vi "Magnet Device (Set).vi"(6 "ISOBUS address":T8=-1 caption="ISOBUS address (-1)", 8 "error in":errorcluster, 10 "Magnet PSU":T3={"Nickname"="", "Bipolar Output"="", "Out Config"="SERS", "Current Limit"=0.0, "AtoB"=0.0, "Inductance"=0.0, "Switch Present"="", "Swh Htr Current"=0.0, "SW VLIM"=0.0, "Ignore Voltage Transient"="", "V Trans Time"=0.0, "Magnet PSU Signals"={"Target Current"=0.0, "Target Field"=0.0, "Target Current Rate"=0.0, "Target Field Rate"=0.0, "Switch Heater Status"="", "Set Switch Heater"="", "PSU Act Stat"="HOLD"}} {"Magnet PSU Signals"."Target Field Rate" min=0.0 max=50.0 step=0.01 format="%#.2f"; "Magnet PSU Signals"."Target Current Rate" min=0.0 max=1200.0 step=0.01 format="%#.2f"; "Magnet PSU Signals"."Target Field" min=-360.0 max=360.0 step=0.01 format="%#.2f"; "Magnet PSU Signals"."Target Current" min=-360.0 max=360.0 step=0.01 format="%#.2f"; "V Trans Time" min=0.0 max=120.0 step=0.01 format="%#.2f"; "SW VLIM" min=0.0 max=12.49 step=0.01 format="%#.2f"; "Swh Htr Current" min=0.0 max=125.0 step=0.01 format="%#.2f"; "Inductance" min=1.0 max=500.0 step=0.01 format="%#.2f"; "AtoB" min=1.0 max=30.0 step=0.01 format="%#.2f"; "Current Limit" min=0.0 max=360.0 step=0.01 format="%#.2f"}, 11 "Mercury Reference In":T9) -> (0 "error out":errorcluster, 2 "Response":T1, 3 "Mercury Reference Out":T9, 4 "Valid?":T2)   [LabVIEW 2013, in "Mercury iXX.lvlib" / "Magnet.lvlib"]
doc: "Set the auxiliary device configuration."
uses:
  Magnet.lvlib
  Mercury iXX.lvlib
  Private/Controls/Command Verbs.ctl
  Controls/Comms Transport Layer.ctl
  Controls/Mercury Reference.ctl
  Controls/Is Valid LED.ctl
  Controls/Response String.ctl
  Controls/ISOBus Address.ctl
  Private/Controls/Query Dynamic Reference.ctl
  Controls/Output Configuration.ctl
  Controls/Switch Heater.ctl
  Controls/PSU Actions.ctl
  Controls/Signals (Set).ctl
  Controls/Device (Set).ctl
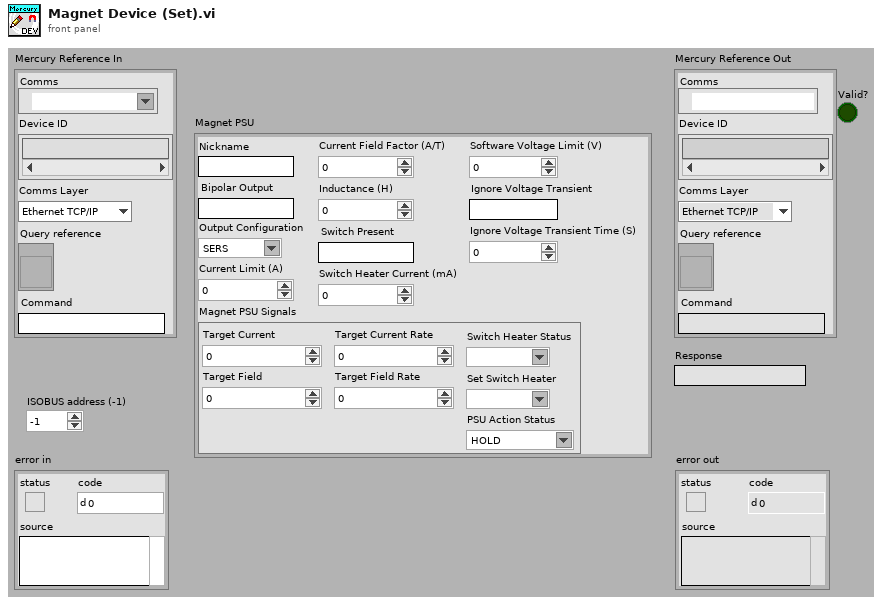
[diagram p1: front panel]
types:
  T1 = typedef "Mercury iXX.lvlib/Response String.ctl" = string
  T2 = typedef "Mercury iXX.lvlib/Is Valid LED.ctl" = bool
  T3 = typedef "Mercury iXX.lvlib/Magnet.lvlib/Device (Set).ctl" = cluster{"Nickname":string, "Bipolar Output":string, "Out Config":T4, "Current Limit":dbl, "AtoB":dbl, "Inductance":dbl, "Switch Present":string, "Swh Htr Current":dbl, "SW VLIM":dbl, "Ignore Voltage Transient":string, "V Trans Time":dbl, "Magnet PSU Signals":T5}
  T4 = typedef "Mercury iXX.lvlib/Magnet.lvlib/Output Configuration.ctl" = string
  T5 = typedef "Mercury iXX.lvlib/Magnet.lvlib/Signals (Set).ctl" = cluster{"Target Current":dbl, "Target Field":dbl, "Target Current Rate":dbl, "Target Field Rate":dbl, "Switch Heater Status":T6, "Set Switch Heater":T6, "PSU Act Stat":T7}
  T6 = typedef "Mercury iXX.lvlib/Magnet.lvlib/Switch Heater.ctl" = string
  T7 = typedef "Mercury iXX.lvlib/Magnet.lvlib/PSU Actions.ctl" = string
  T8 = typedef "Mercury iXX.lvlib/ISOBus Address.ctl" = i32
  T9 = typedef "Mercury iXX.lvlib/Mercury Reference.ctl" = cluster{"Comms":refnum<visa-resource-name>, "Device ID":string[], "Comms Layer":T10, "Command":string, "Query reference":T11}
  T10 = typedef "Mercury iXX.lvlib/Comms Transport Layer.ctl" = enum16{"Ethernet TCP/IP", "USB", "ISOBus - RS-232", "GPIB"}
  T11 = typedef "Mercury iXX.lvlib/Query Dynamic Reference.ctl" = refnum<vi>
  T12 = typedef "Mercury iXX.lvlib/Command Verbs.ctl" = string
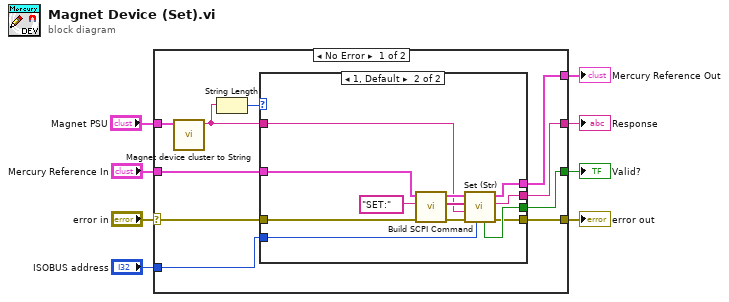
[diagram p0: block diagram]
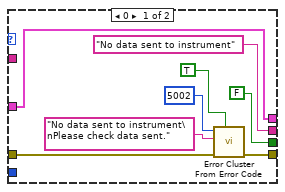
[diagram p2: hidden frame]
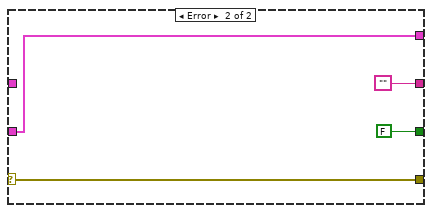
[diagram p3: hidden frame]
diagram:
  n1 = case shown="No Error" "error in" {
    selector: "error in" -> [w18 w41]
    tunnel: "Mercury Reference In" -> [w14 w42]
    tunnel: [w15 w42] -> w7
    tunnel: [w16 w41] -> w6
    tunnel: "ISOBUS address" -> [w17 _]
    tunnel: [w9 ""] -> w2
    tunnel: [w10 FALSE ("Valid?")] -> w3
    tunnel: "Magnet PSU" -> [w12 _]
    frame No Error {
      n2 = call "Magnet device cluster to String.vi"("Magnet PSU"=w12) -> ("Data to send"=w11:string)  [unwired: 10 out]
      n3 = String Length(string=w11) -> (length=w13:i32)
      n4 = case shown="1, Default" w13 {
        tunnel: ["No data sent to instrument" ("Data") w38] -> w9
        tunnel: [FALSE ("Valid?") w37] -> w10
        tunnel: w14 -> [w26 w29]
        tunnel: w17 -> [_ w35]
        tunnel: w18 -> [w24 w28]
        tunnel: [w25 w34] -> w16
        tunnel: [w26 w36] -> w15
        tunnel: w11 -> [_ w30]
        frame 0 {
          n5 = call <vilib>:"Error Cluster From Error Code.vi"("show call chain? (False)"=TRUE, "error in (no error)"=w24, "error message (\"\")"="No data sent to instrument\nPlease check data sent." ("error message (\"\")"), "error code (0)"=5002) -> ("error out"=w25:errorcluster)  [unwired: 5 out]
        }
        frame 1, Default {
          n6 = call "Build SCPI Command.vi"("error in"=w28, "Verb"=T12 "SET:", "Mercury Reference In"=w29) -> ("error out"=w31:errorcluster, "SCPI Message(s)"=w32:string[], "Mercury Reference Out"=w33:T9)  [unwired: 1 in, 5 out]
          n7 = call "Set (Str).vi"("ISOBUS address"=w35, "error in"=w31, "Command Value (Str)"=w30, "SCPI Message(s)"=w32, "Mercury Reference In"=w33) -> ("error out"=w34:errorcluster, "Response"=w38:T1, "Mercury Reference Out"=w36:T9, "Valid?"=w37:T2)  [unwired: 3 out]
        }
      }
    }
    frame Error {
    }
  }
  "Mercury Reference Out" <- w7
  "error out" <- w6
  "Valid?" <- w3
  "Response" <- w2
